vi "Monitor.vi"() -> ()   [LabVIEW 2016]
uses:
  Typedefs/Monitor Data Cluster.ctl
  <vilib>/Platform/TimedLoop/XDataNode/timing_clust.ctl
  <vilib>/Platform/TimedLoop/XDataNode/nitl_modes.ctl
  <vilib>/Platform/TimedLoop/XDataNode/wakeup.ctl
  <vilib>/rvi/Emulation/niFpgaSctlEmulationGetInTimedLoop.vi
  <vilib>/rvi/Emulation/niFpgaEmulationReportErrorSimple.vi
  <vilib>/rvi/Emulation/niFpgaGetClockAttributes.vi
  <vilib>/rvi/Emulation/niFpgaCriticalErrorInLSC.vi
  <vilib>/Platform/TimedLoop/XDataNode/XDataNode.xnode
  <vilib>/Platform/TimedLoop/XDataNode/XDNodeRunTimeDep.lvlib
panel:
  out "Overflow?":bool
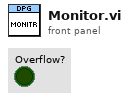
[diagram p1: front panel]
types:
  T1 = typedef "Monitor Data Cluster.ctl" = cluster{"Tick Count":u32, "Data to Host":u64, "Write FIFO?":bool, "Enable Monitor?":bool}
  T2 = typedef "XDNodeRunTimeDep.lvlib/timing_clust.ctl" = cluster{"Expected End [f-1]":u64, "Actual End [f-1]":u64, "Finished Late? [f-1]":bool, "Expected End [i-1]":u64, "Actual End [i-1]":u64, "Finished Late? [i-1]":bool, "Expected Start [i]":u64, "Actual Start [i]":u64, "Expected Start [f]":u64, "Actual Start [f]":u64, "Source Name":string, "Structure Name":string, "Period":i64, "Deadline":i64, "Offset":i64, "Start":i64, "Priority":i32, "Timeout":i32, "Mode":T3, "Wakeup Reason":T4, "Error":errorcluster, "Source Type":string, "Secondary Source Type":string, "Global End Time":u64, "Global Start Time":u64, "Frame Duration":u64, "Iteration Duration":u64, "Assigned CPU":i32, "I/O Scan Engine Mode":u32}
  T3 = typedef "XDNodeRunTimeDep.lvlib/nitl_modes.ctl" = enum32{"No Change", "Process missed periods, maintain original phase", "Discard missed periods, maintain original phase", "Process missed periods, ignore original phase", "Discard missed periods, ignore original phase"}
  T4 = typedef "XDNodeRunTimeDep.lvlib/wakeup.ctl" = enum32{"Normal", "Aborted", "Asynchronous wakeup", "Timing source error", "Timed loop error", "Timeout"}
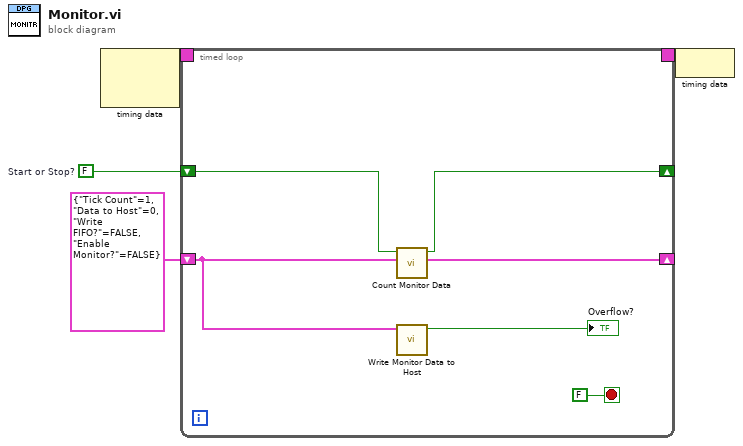
[diagram p0: block diagram]
diagram:
  w1 = FALSE  # Start or Stop?
  n1 = node-c288() -> (w4:T2)  [unwired: 2 in]
  n2 = timed-loop {
    timing: w4 -> [_]
    timing-out: [_] -> w3
    shift-right: [w10] -> _
    shift-left: T1 {"Tick Count"=1, "Data to Host"=0, "Write FIFO?"=FALSE, "Enable Monitor?"=FALSE} ("Monitor Data Cluster") -> [w7]
    shift-right: [w6] -> _
    shift-left: w1 -> [w8]
    stop <- FALSE stop-if-true
    n3 = call "Count Monitor Data.vi"("Monitor Data Cluster in"=w7, "Start or Stop Enable?"=w8) -> ("Monitor Data Cluster out"=w10:T1, "Enable?"=w6:bool)  [unwired: 8 in]
    n4 = call "Write Monitor Data to Host.vi"("Monitor Data Cluster"=w7) -> ("Overflow?"=→"Overflow?":bool)  [unwired: 10 in]
  }
  n5 = node-c288(w3) -> ()
